vi "niRFUtil FWK Compute Minimum Quanta.vi"(8 "error in (no error)":errorcluster, 10 "Offset Frequency (Hz)":dbl=1000.0 format="%^.2e", 11 "Minimum Frequency Quanta (-1 Hz = Auto)":dbl=-1.0) -> (0 "error out":errorcluster, 3 "Actual Frequency Quanta (Hz)":dbl=1000.0 format="%^.2e")   [LabVIEW 2015, in "niRFUtil.lvlib"]
doc: "(c) Copyright 2006, National Instruments, Inc. This VI may not be duplicated, sold, or distributed without written consent from National Instruments."
uses:
  niRFUtil.lvlib
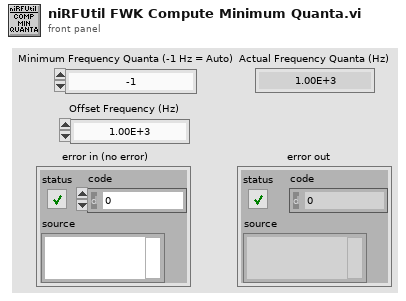
[diagram p1: front panel]
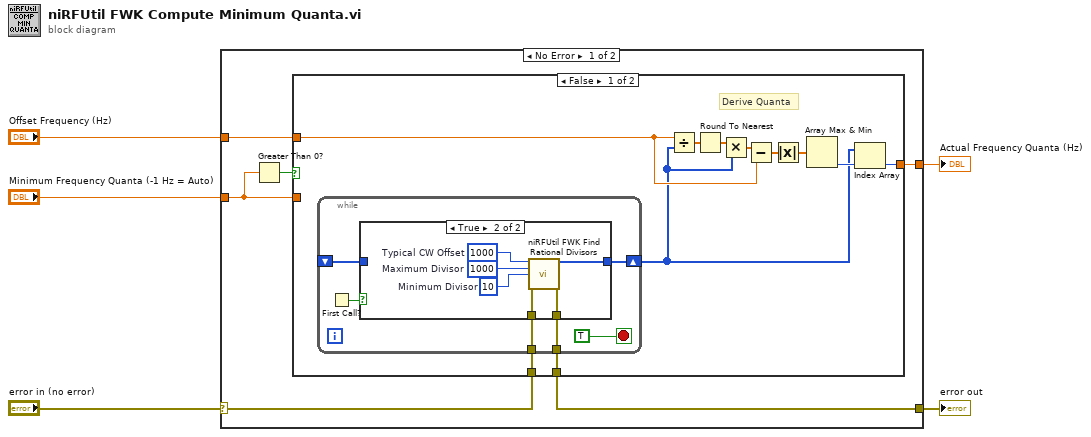
[diagram p0: block diagram]
diagram:
  n1 = case shown="No Error" "error in (no error)" {
    selector: "error in (no error)" -> [w7 w39]
    tunnel: [w6 w39] -> w4
    tunnel: "Offset Frequency (Hz)" -> [w11 _]
    tunnel: [w10 _] -> w2
    tunnel: "Minimum Frequency Quanta (-1 Hz = Auto)" -> [w9 _]
    frame No Error {
      n2 = Greater Than 0?(x=w9) -> (x > 0?=w8:bool)
      n3 = case shown="False" w8 {
        tunnel: w11 -> [w22 _]
        tunnel: w9 -> [_ w38]
        tunnel: [w21 w38] -> w10
        tunnel: w7 -> [w14 w37]
        tunnel: [w13 w37] -> w6
        frame False {
          # "Derive Quanta"
          n4 = while {
            tunnel: w14 -> [w28]
            tunnel: [w27] -> w13
            shift-right: [w25] -> w12
            shift-left: _ -> [w24]
            stop <- TRUE stop-if-true
            n5 = First Call?() -> (First Call?: T/F=w26:bool)
            n6 = case shown="True" w26 {
              tunnel: w28 -> [w29 w36]
              tunnel: [w29 w35] -> w27
              tunnel: [w30 w31] -> w25
              tunnel: w24 -> [w30 _]
              frame False {
              }
              frame True {
                w32 = 10  # Minimum Divisor
                w33 = 1000  # Maximum Divisor
                w34 = 1000  # Typical CW Offset
                n7 = call "niRFUtil FWK Find Rational Divisors.vi"("Number"=w34, "Maximum Divisor"=w33, "Minimum Divisor"=w32, "error in (no error)"=w36) -> ("Divisors"=w31:i32[], "error out"=w35:errorcluster)  [unwired: 10 out]
              }
            }
          }
          n8 = Divide(x=w22, y=w12) -> (x/y=w18:dbl[])
          n9 = Round To Nearest(number=w18) -> (nearest integer value=w17:dbl[])
          n10 = Multiply(x=w17, y=w12) -> (x*y=w16:dbl[])
          n11 = Subtract(x=w16, y=w22) -> (x-y=w15:dbl[])
          n12 = Absolute Value(x=w15) -> (abs(x)=w19:dbl[])
          n13 = Array Max & Min(array=w19) -> (min index (indices)=w20:i32)  [unwired: 3 out]
          n14 = Index Array(array=w12, index=w20) -> (element=w21:i32)
        }
        frame True {
          # "Use requested quanta"
        }
      }
    }
    frame Error {
    }
  }
  "Actual Frequency Quanta (Hz)" <- w2
  "error out" <- w4
